vi "Pre Launch Init.vi"(11 "Arduino_Stepper in":refnum<class "Arduino_Stepper_UI.lvclass">) -> (0 "error out":errorcluster, 3 "Arduino_Stepper out":refnum<class "Arduino_Stepper_UI.lvclass">)   [LabVIEW 2023, in "Arduino_TranslationStage_UI.lvlib" / "Arduino_Stepper_UI.lvclass"]
doc: "(<B>Filename</B>: Actor Framework.lvlib:Actor.lvclass:Pre Launch Init.vi)\n\nDefines behavior that occurs after the Launch Nested Actor method is invoked but before the actor's Actor Core method begins running.\n\nBy default, this method does nothing. A descendant class may override it to define behavior."
uses:
  Arduino_Stepper_UI.lvclass
  <vilib>/ActorFramework/Actor/Actor.lvclass
  TranslationStage_UI/TranslationStage_UI/StageMoveDone_For_UI.ctl
  typedefs/typedefs.lvlib
panel:
  in  "Variant":variant
  in  "Registers":u16[][](array[numeric])
  in  "Positions":T1={"CH1 Pos"=0.0, "CH2 Pos"=0.0, "CH3 Pos"=0.0, "CH4 Pos"=0.0, "Home?"=TRUE}
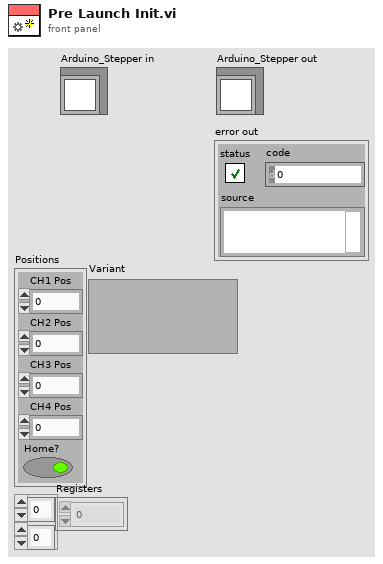
[diagram p1: front panel]
types:
  T1 = typedef "typedefs.lvlib/StageMoveDone_For_UI.ctl" = cluster{"CH1 Pos":sgl, "CH2 Pos":dbl, "CH3 Pos":dbl, "CH4 Pos":dbl, "Home?":bool}
  T2 = cluster{"Scanning Done":bool, "Axis":enum16{"X", "Y", "Z", "HOM"}}
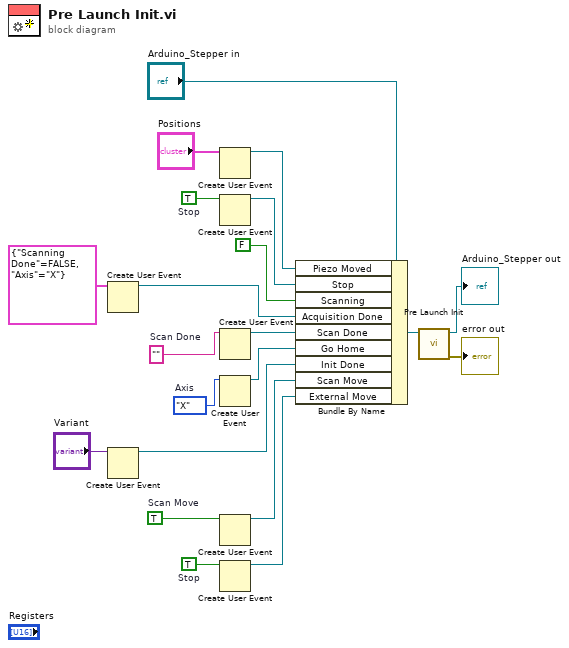
[diagram p0: block diagram]
diagram:
  w2 = TRUE  # Stop
  w4 = TRUE  # Scan Move
  w9 = enum16{"X", "Y", "Z", "HOM"}."X"  # Axis
  w15 = ""  # Scan Done
  w18 = TRUE  # Stop
  n1 = Create User Event(user event datatype=T2 {"Scanning Done"=FALSE, "Axis"=enum."X"} ("Acq Done Data")) -> (user event=w16:refnum<user-event>)  [unwired: 1 in, 1 out]
  n2 = Create User Event(user event datatype="Variant") -> (user event=w7:refnum<user-event>)  [unwired: 1 in, 1 out]
  n3 = Create User Event(user event datatype="Positions") -> (user event=w13:refnum<user-event>)  [unwired: 1 in, 1 out]
  n4 = Create User Event(user event datatype=w18) -> (user event=w19:refnum<user-event>)  [unwired: 1 in, 1 out]
  n5 = Create User Event(user event datatype=w15) -> (user event=w14:refnum<user-event>)  [unwired: 1 in, 1 out]
  n6 = Create User Event(user event datatype=w9) -> (user event=w10:refnum<user-event>)  [unwired: 1 in, 1 out]
  n7 = Create User Event(user event datatype=w4) -> (user event=w3:refnum<user-event>)  [unwired: 1 in, 1 out]
  n8 = Create User Event(user event datatype=w2) -> (user event=w1:refnum<user-event>)  [unwired: 1 in, 1 out]
  n9 = Bundle By Name(cluster="Arduino_Stepper in", "Piezo Moved"=w13, "Stop"=w19, "Scanning"=FALSE ("Cam Connected"), "Acquisition Done"=w16, "Scan Done"=w14, "Go Home"=w10, "Init Done"=w7, "Scan Move"=w3, "External Move"=w1) -> (w5:refnum<class "Arduino_Stepper_UI.lvclass">)
  n10 = call-parent "Pre Launch Init.vi"("Actor in"=w5) -> ("error out"=→"error out":errorcluster, "Actor out"=→"Arduino_Stepper out":refnum<class "Arduino_Stepper_UI.lvclass">)  [unwired: 9 in]
